vi "Edit Line.vi"(8 "error in":errorcluster, 10 "Line Name":string, 11 "References":T1) -> (0 "error out":errorcluster, 2 "change?":bool)   [LabVIEW 2014, in "tag bus configurable plugin editor node.lvclass"]
uses:
  tag bus configurable plugin editor node.lvclass
  Table Manager/object ref.ctl
  Configuration Editor/Classes/Engine Parent/Engine Parent Editor Node.lvclass
  Configuration Editor/Classes/Module editor node/module editor node.lvclass
  module/configuration/tag bus configurable plugin module configuration.lvclass
  module/configuration/tag bus configurable plugin module configuration.lvclass/tag bus configurable plugin module configuration.ctl
  <vilib>/NI/Configuration Framework/serializable configuration/NISE_CEF_serializable configuration.lvclass/NISE_CEF_serializable configuration.ctl
  <vilib>/Utility/LVClass/Get LV Class Name.vi
  <vilib>/NI/Configuration Framework/error generator/NISE_error generator.vi
  <vilib>/NI/Tag Bus Module Framework/channel/TBM channel.lvclass
  <vilib>/NI/Configuration Framework/serializable configuration/NISE_CEF_serializable configuration.lvclass
  Table Manager/Table Manager.lvclass
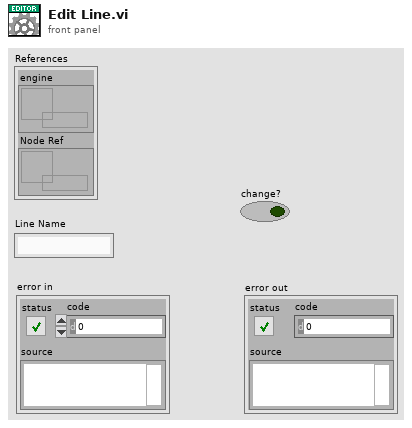
[diagram p1: front panel]
types:
  T1 = typedef "Table Manager.lvlib/Table Manager.lvclass/object ref.ctl" = cluster{"engine":refnum<data-value>, "Node Ref":refnum<data-value>}
  T2 = typedef "tag bus configurable plugin module configuration.lvclass/Line.ctl" = cluster{"channel":refnum<class "TBM channel.lvclass">}
  T3 = typedef "tag bus configurable plugin editor node.lvclass/Mappings.ctl" = cluster{"Line":T2, "Maps":T4[]}
  T4 = typedef "tag bus configurable plugin editor node.lvclass/Map.ctl" = cluster{"channel":refnum<class "TBM channel.lvclass">, "tag name":string}
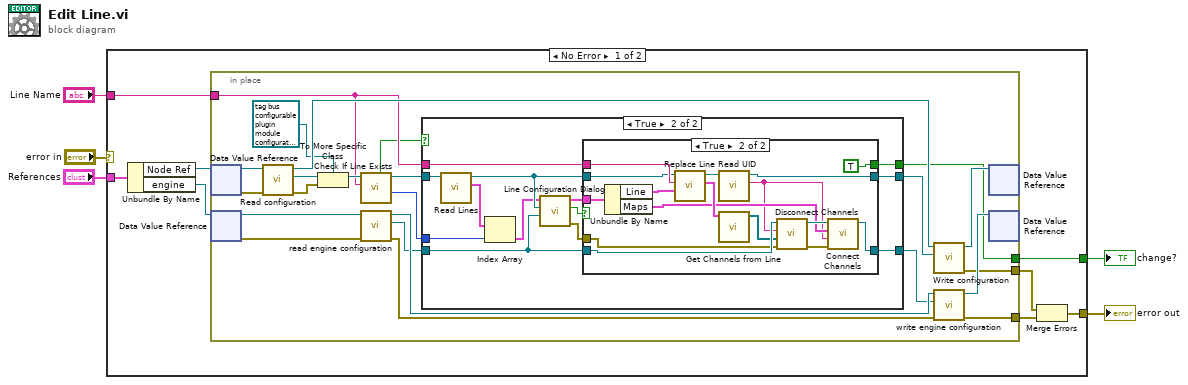
[diagram p0: block diagram]
diagram:
  n1 = case shown="No Error" "error in" {
    selector: "error in" -> [_ w70]
    tunnel: "References" -> [w11 _]
    tunnel: "Line Name" -> [w10 _]
    tunnel: [w7 w70] -> w2
    tunnel: [w6 _] -> w1
    frame No Error {
      n2 = Unbundle By Name(w11) -> ("Node Ref"=w13:refnum<data-value>, "engine"=w12:refnum<data-value>)
      n3 = in-place {
        in-place-border: [w17] -> w9
        in-place-border: [w33] -> w8
        in-place-border: [w16] -> w6
        in-place-border: w10 -> [w22]
        n4 = in-place-dvr #1(w13) -> (w29:refnum<class "module editor node.lvclass">, w23:errorcluster)
        n5 = in-place-dvr #2(w12) -> (w36:refnum<class "Engine Parent Editor Node.lvclass">, w35:errorcluster)
        n6 = call-dynamic "Read configuration.vi"("error in"=w23, "NISE_CEF_serializable node in"=w29) -> ("error out"=w26:errorcluster, "configuration"=w27:refnum<class "NISE_CEF_serializable configuration.lvclass">, "NISE_CEF_serializable node out"=w28:refnum<class "module editor node.lvclass">)  [unwired: 7 in]
        n7 = To More Specific Class(target class=refnum<class "tag bus configurable plugin module configuration.lvclass"> refnum ("tag bus configurable plugin module configuration"), reference=w27, error in=w26) -> (specific class reference=w24:refnum<class "tag bus configurable plugin module configuration.lvclass">)  [unwired: 1 out]
        n8 = call-dynamic "Check If Line Exists.vi"("name to locate"=w22, "tag bus configurable plugin module configuration in"=w24) -> ("index"=w19:i32, "tag bus configurable plugin module configuration out"=w20:refnum<class "tag bus configurable plugin module configuration.lvclass">, "found?"=w14:bool)  [unwired: 5 in, 2 out]
        n9 = call "read engine configuration.vi"("error in"=w35, "Engine Parent Editor Node in"=w36) -> ("error out"=w31:errorcluster, "engine configuration"=w18:refnum<class "engine configuration.lvclass">, "Engine Parent Editor Node out"=w32:refnum<class "Engine Parent Editor Node.lvclass">)  [unwired: 7 in]
        n10 = case shown="True" w14 {
          tunnel: w20 -> [w38 w49]
          tunnel: w18 -> [w37 w39]
          tunnel: w22 -> [_ w51]
          tunnel: [w38 w43] -> w21
          tunnel: w19 -> [_ w46]
          tunnel: [_ w41] -> w16
          tunnel: [w37 w40] -> w15
          frame False {
          }
          frame True {
            n11 = call "Read Lines.vi"("tag bus configurable plugin module configuration in"=w49) -> ("Lines"=w47:T2[], "tag bus configurable plugin module configuration out"=w48:refnum<class "tag bus configurable plugin module configuration.lvclass">)  [unwired: 8 in, 1 out]
            n12 = Index Array(array=w47, index=w46) -> (element=w45:T2)
            n13 = call "Line Configuration Dialog.vi"("engine configuration in"=w39, "tag bus configurable plugin module configuration"=w48, "Line"=w45) -> ("error out"=w50:errorcluster, "changed"=w42:bool, "Mappings out"=w44:T3)  [unwired: 5 in, 1 out]
            n14 = case shown="True" w42 {
              tunnel: w51 -> [_ w69]
              tunnel: w39 -> [w52 w68]
              tunnel: w50 -> [_ w67]
              tunnel: w48 -> [w53 w63]
              tunnel: w44 -> [_ w62]
              tunnel: [w53 w60] -> w43
              tunnel: [_ TRUE ("change?")] -> w41
              tunnel: [w52 w54] -> w40
              frame False {
              }
              frame True {
                n15 = Unbundle By Name(w62) -> ("Line"=w61:T2, "Maps"=w57:T4[])
                n16 = call "Replace Line.vi"("New Line"=w61, "Line Name"=w69, "tag bus configurable plugin module configuration in"=w63) -> ("Old Line"=w65:T2, "tag bus configurable plugin module configuration out"=w66:refnum<class "tag bus configurable plugin module configuration.lvclass">)  [unwired: 6 in, 1 out]
                n17 = call <vilib>:"Read UID.vi"("configuration in"=w66) -> ("instance id"=w56:string, "configuration out"=w60:refnum<class "tag bus configurable plugin module configuration.lvclass">)  [unwired: 8 in, 1 out]
                n18 = call "Get Channels from Line.vi"("Line"=w65) -> ("Array"=w64:refnum<class "TBM channel.lvclass">[])  [unwired: 10 in]
                n19 = call "Disconnect Channels.vi"("error in (no error)"=w67, "Deleted Channels"=w64, "instance id"=w56, "engine configuration in"=w68) -> ("error out"=w58:errorcluster, "engine configuration out"=w59:refnum<class "engine configuration.lvclass">)  [unwired: 6 in]
                n20 = call "Connect Channels.vi"("error in (no error)"=w58, "instance id"=w56, "Maps"=w57, "engine configuration in"=w59) -> ("engine configuration out"=w54:refnum<class "engine configuration.lvclass">)  [unwired: 6 in, 1 out]
              }
            }
          }
        }
        n21 = call-dynamic "Write configuration.vi"("configuration"=w21, "NISE_CEF_serializable node in"=w28) -> ("error out"=w17:errorcluster, "NISE_CEF_serializable node out"=w30:refnum<class "module editor node.lvclass">)  [unwired: 8 in]
        n22 = call "write engine configuration.vi"("error in"=w31, "engine configuration"=w15, "Engine Parent Editor Node in"=w32) -> ("error out"=w33:errorcluster, "Engine Parent Editor Node out"=w34:refnum<class "Engine Parent Editor Node.lvclass">)  [unwired: 7 in]
        n23 = in-place-dvr #1(w30) -> ()  [unwired: 2 out]
        n24 = in-place-dvr #2(w34) -> ()  [unwired: 2 out]
      }
      n25 = Merge Errors(w9, w8) -> (w7:errorcluster)
    }
    frame Error {
    }
  }
  "change?" <- w1
  "error out" <- w2
